vi "secret_key.vi"(11 "creds":path=path "/Users/milandahal/Documents/GitHub/Onshape/python/creds.json") -> (0 "output cluster":T1)   [LabVIEW 2019]
panel:
  in  "input":T1={"Date"="Thu, 12  Mar 2020 17:36:12 GMT", "On-Nonce"="2wnETveaz9elinoAv7Quei4r", "ctype"="application/json", "path"="/api/documents", "method"="get", "Authorization"="On ktems66AXXcKmV1AjxwpmVkx:HmacSHA256:q+pYGzGt3CZyb2jkZokip3yYBD8R7CzNT+OBIk9yl5c=", "Accept"="application/json", "User-Agent"="Onshape Python Sample App", "Content-Type"="application/json", "secret_key"="", "access_key"="", "stack"="https://rogers.onshape.com", "payload"=""}
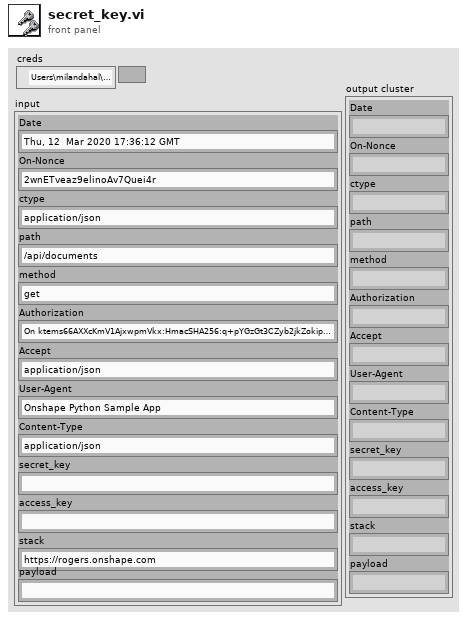
[diagram p1: front panel]
types:
  T1 = cluster{"Date":string, "On-Nonce":string, "ctype":string, "path":string, "method":string, "Authorization":string, "Accept":string, "User-Agent":string, "Content-Type":string, "secret_key":string, "access_key":string, "stack":string, "payload":string}
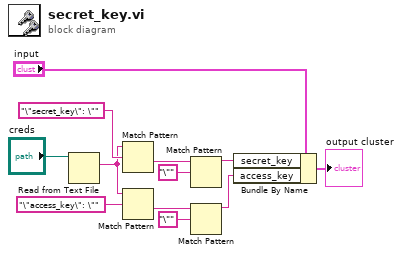
[diagram p0: block diagram]
diagram:
  n1 = Read from Text File(file (use dialog)="creds") -> (text=w5:string)  [unwired: 3 in, 3 out]
  n2 = Match Pattern(string=w5, regular expression="\"secret_key\": \"") -> (after substring=w9:string)  [unwired: 1 in, 3 out]
  n3 = Match Pattern(string=w5, regular expression="\"access_key\": \"") -> (after substring=w7:string)  [unwired: 1 in, 3 out]
  n4 = Match Pattern(string=w9, regular expression="\"") -> (before substring=w4:string)  [unwired: 1 in, 3 out]
  n5 = Match Pattern(string=w7, regular expression="\"") -> (before substring=w3:string)  [unwired: 1 in, 3 out]
  n6 = Bundle By Name(cluster="input", "secret_key"=w4, "access_key"=w3) -> (→"output cluster":T1)
